vi "RunTest3.vi"(8 "error in (no error)":errorcluster, 11 "Prueba01 in":refnum<class "Prueba01.lvclass">) -> (0 "error out":errorcluster, 2 "resultado":string, 3 "Prueba01 out":refnum<class "Prueba01.lvclass">)   [LabVIEW 2019]
uses:
  Prueba01.lvclass
panel:
  in  "Tab Control":enum32{"externo", "interno"}(tab)
  out "max_tol_ajuste_ext":dbl
  out "Nivel_externo":dbl
  in  "generar":bool
  out "frecuencia":dbl
  out "cumple":bool
  out "no_cumple":bool
  out "frec_ref":dbl
  out "nivel_ref":dbl
  in  "señal_antes_ajuste":dbl
  out "error_ext":dbl
  out "inc_extend":dbl
  in  "seguir":bool
  out "voltaje":dbl
  out "frecuencia 2":dbl
  out "tipo generador":string
  out "max_tol_ajuste_int":dbl
  in  "Nivel_interno":dbl
  out "frecuencia_int":dbl
  out "cumple_int":bool
  out "no_cumple_int":bool
  out "frec_ref_int":dbl
  out "nivel_ref_int":dbl
  in  "señal_antes_ajuste_int":dbl
  out "error_ext_int":dbl
  out "inc_extend_int":dbl
  in  "seguir_int":bool
  out "tipo gen_int":string
  # "Elección Señal de Referencia \nsegún marca y modelo de sonómetro"
  # "Cumple"
  # "No Cumple"
  # "Máxima Tolerancia de Ajuste"
  # "Frecuencia"
  # "Nivel"
  # "Frecuencia Señal de Referencia [Hz]"
  # "Nivel de Señal de Referencia [dB] (a)"
  # "Nivel de señal medida antes de ajuste [dB] (b)"
  # "Error [dB]"
  # "Incertidumbre Expandida ± [dB] (k=2)"
  # "1. Indicación a la frecuencia de comprobación. IEC 61672-3: 2006 Cláusula 9"
  # "Monitoreo"
  # "Frecuencia"
  # "Hz"
  # "Voltaje"
  # "V"
  # "Elección Señal de Referencia \nsegún marca y modelo de sonómetro"
  # "Máxima Tolerancia de ajuste"
  # "Cumple"
  # "No Cumple"
  # "Frecuencia"
  # "Nivel"
  # "Frecuencia Señal de Referencia [Hz]"
  # "Nivel de Señal de Referencia [dB] (a)"
  # "Nivel de señal medida antes de ajuste [dB] (b)"
  # "Error [dB]"
  # "Incertidumbre Expandida ± [dB] (k=2)"
  # "1. Indicación a la frecuencia de comprobación. IEC 61672-3: 2006 Cláusula 9"
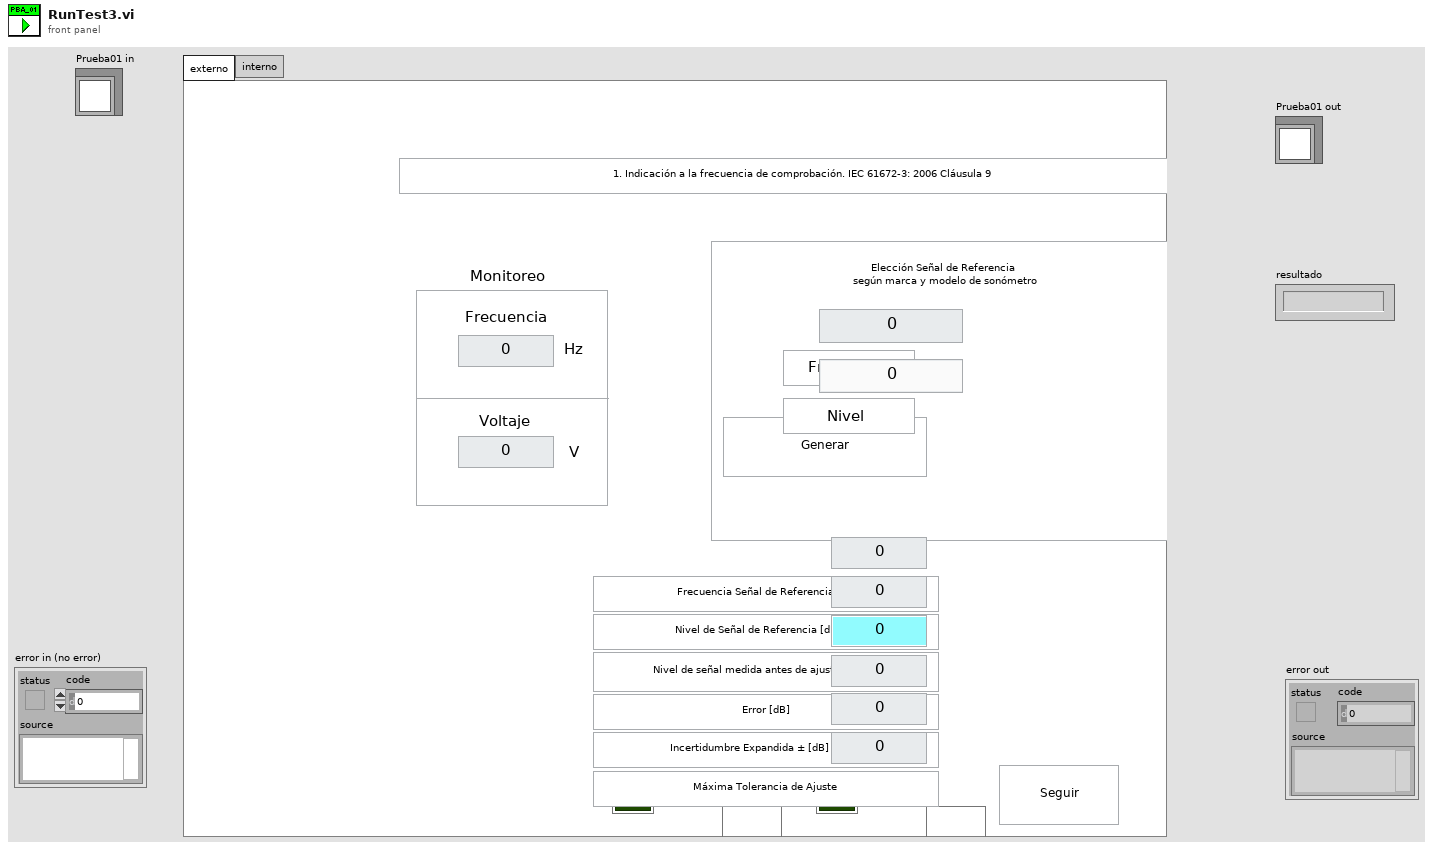
[diagram p1: front panel]
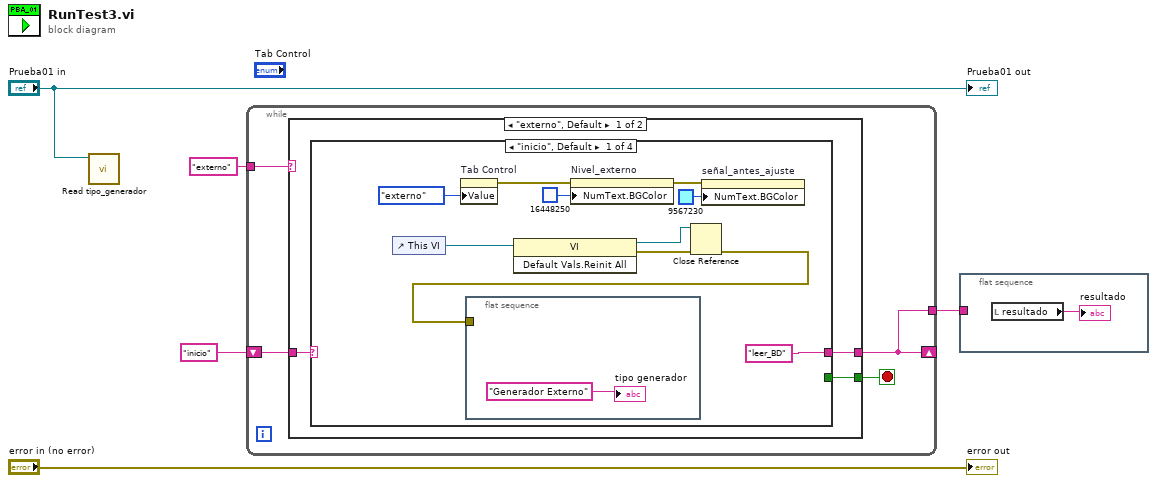
[diagram p0: block diagram]
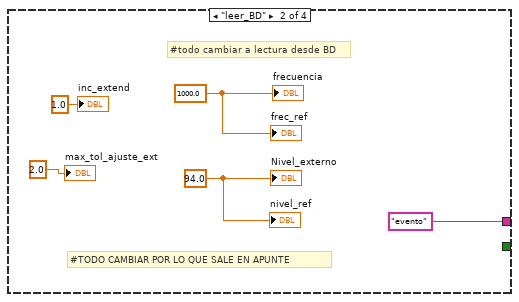
[diagram p2: hidden frame]
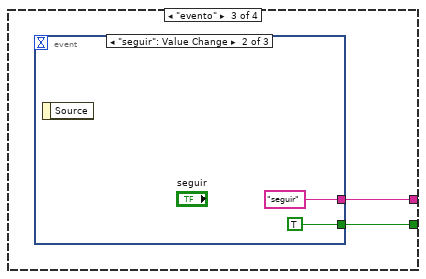
[diagram p3: hidden frame]
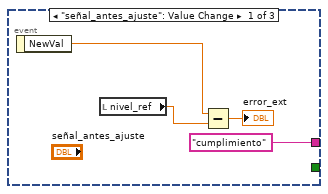
[diagram p4: hidden frame]
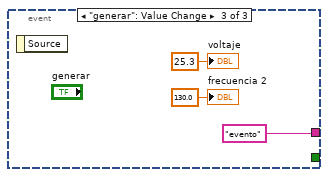
[diagram p5: hidden frame]
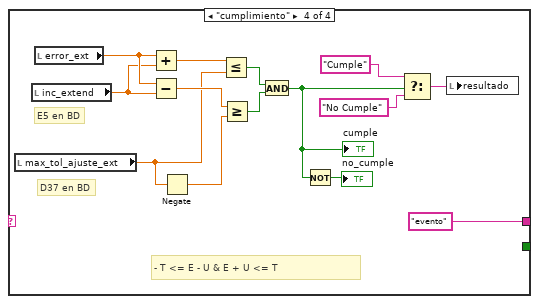
[diagram p6: hidden frame]
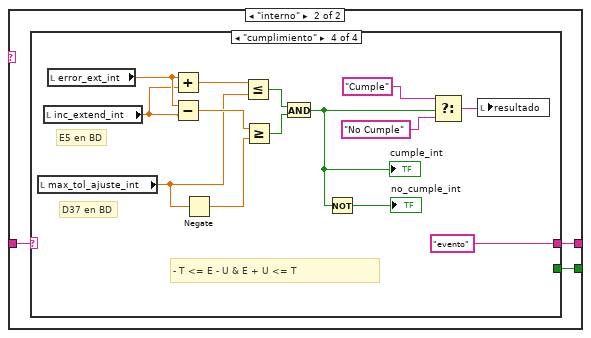
[diagram p7: hidden frame]
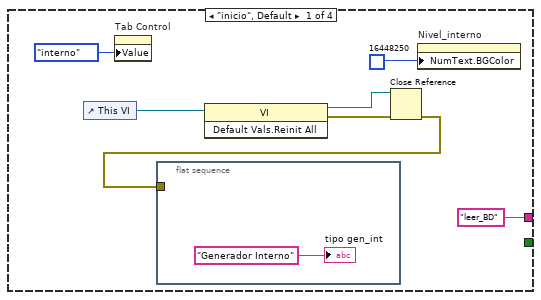
[diagram p8: hidden frame]
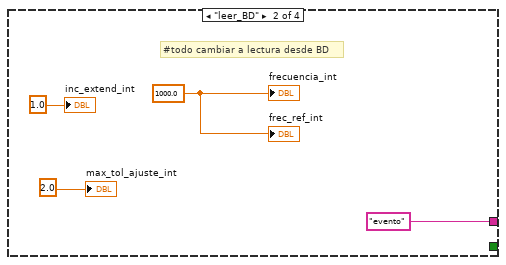
[diagram p9: hidden frame]
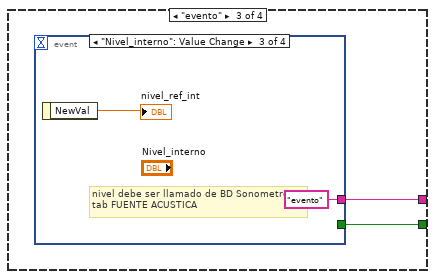
[diagram p10: hidden frame]
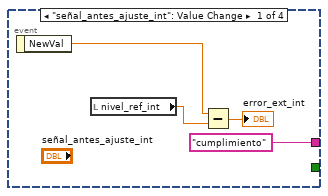
[diagram p11: hidden frame]
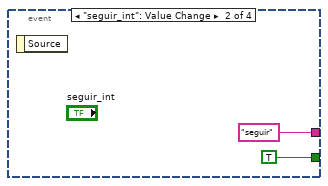
[diagram p12: hidden frame]
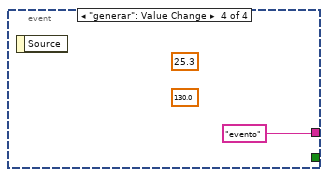
[diagram p13: hidden frame]
diagram:
  n1 = call-dynamic "Read tipo_generador.vi"("Prueba01 in"="Prueba01 in") -> ()  [unwired: 8 in, 3 out]
  n2 = while {
    shift-right: [w6] -> _
    shift-left: "inicio" -> [w9]
    tunnel: "externo" ("tipo_generador") -> [w7]
    tunnel: [w6] -> w2
    stop <- w8 stop-if-true
    n3 = case shown="\"externo\", Default" w7 {
      tunnel: w9 -> [w12 w56]
      tunnel: [w11 w55] -> w8
      tunnel: [w10 w54] -> w6
      frame "externo", Default {
        n4 = case shown="\"inicio\", Default" w12 {
          tunnel: ["leer_BD" "evento" w30 "evento"] -> w10
          tunnel: [_ _ w29 _] -> w11
          frame "inicio", Default {
            n5 = control-ref of="This VI"() -> (w20:refnum<vi>)
            n6 = property on="Tab Control" class="TabCtl (strict)"("Value"=enum32{"externo", "interno"}."externo" ("Tab Control")) -> (error out=w15:errorcluster)  [unwired: 2 in, 1 out]
            n7 = flat-sequence {
              tunnel: w18 -> [_]
              frame #0 {
                "tipo generador" <- "Generador Externo" ("Generador")
              }
            }
            n8 = invoke class="VI" method="Default Vals.Reinit All"(reference=w20) -> (reference out=w21:refnum<vi>, error out=w22:errorcluster)  [unwired: 2 in, 1 out]
            n9 = property on="Nivel_externo" class="DigNum (strict)"(error in=w15, "NumText.BGColor"=u32 16448250) -> (error out=w14:errorcluster)  [unwired: 1 in, 1 out]
            n10 = Close Reference(reference=w21, error in (no error)=w22) -> (error out=w18:errorcluster)
            n11 = property on="señal_antes_ajuste" class="DigNum (strict)"(error in=w14, "NumText.BGColor"=u32 9567230) -> ()  [unwired: 1 in, 2 out]
          }
          frame "leer_BD" {
            w26 = 94.0 ("Nivel_externo")
            w27 = 1000.0 ("frecuencia")
            # "#TODO CAMBIAR POR LO QUE SALE EN APUNTE"
            # "#todo cambiar a lectura desde BD"
            "frecuencia" <- w27
            "frec_ref" <- w27
            "Nivel_externo" <- w26
            "nivel_ref" <- w26
            "inc_extend" <- 1.0 ("incertidumbre")
            "max_tol_ajuste_ext" <- 2.0 ("Tolerancia")
          }
          frame "evento" {
            n12 = event shown="[1] \"seguir\": Value Change" {
              selector: _ -> [_ _ _]
              dyn-events: _ -> [_ _ _]
              timeout: _ -> [_ _ _]
              tunnel: ["cumplimiento" "seguir" "evento"] -> w30
              tunnel: [_ TRUE _] -> w29
              event "señal_antes_ajuste": Value Change {
                n13 = event-data() -> ("NewVal"=w32:dbl)  [unwired: 1 in]
                n14 = local read "nivel_ref"() -> (w31:dbl)
                n15 = Subtract(x=w32, y=w31) -> (x-y=→"error_ext":dbl)
              }
              event "seguir": Value Change {
                n16 = event-data() -> ()  [unwired: 1 in, 1 out]
              }
              event "generar": Value Change {
                n17 = event-data() -> ()  [unwired: 1 in, 1 out]
                "frecuencia 2" <- 130.0 ("frecuencia")
                "voltaje" <- 25.3 ("voltaje")
              }
            }
          }
          frame "cumplimiento" {
            # "D37 en BD"
            # "- T <= E - U & E + U <= T"
            # "E5 en BD"
            n18 = local read "max_tol_ajuste_ext"() -> (w40:dbl)
            n19 = local read "inc_extend"() -> (w43:dbl)
            n20 = local read "error_ext"() -> (w49:dbl)
            n21 = Add(x=w49, y=w43) -> (x+y=w48:dbl)
            n22 = Subtract(x=w49, y=w43) -> (x-y=w45:dbl)
            n23 = Negate(x=w40) -> (-x=w42:dbl)
            n24 = Less Or Equal?(x=w48, y=w40) -> (x <= y?=w47:bool)
            n25 = Greater Or Equal?(x=w45, y=w42) -> (x >= y?=w46:bool)
            n26 = And(x=w47, y=w46) -> (x .and. y?=w44:bool)
            "cumple" <- w44
            n27 = Not(x=w44) -> (.not. x?=→"no_cumple":bool)
            n28 = Select(t="Cumple", s=w44, f="No Cumple") -> (s? t:f=w41:string)
            n29 = local write "resultado"(w41) -> ()
          }
        }
      }
      frame "interno" {
        n30 = case shown="\"cumplimiento\"" w56 {
          tunnel: ["leer_BD" "evento" w70 "evento"] -> w54
          tunnel: [_ _ w69 _] -> w55
          frame "inicio", Default {
            n31 = control-ref of="This VI"() -> (w61:refnum<vi>)
            n32 = property on="Tab Control" class="TabCtl (strict)"("Value"=enum32{"externo", "interno"}."interno" ("Tab Control")) -> ()  [unwired: 2 in, 2 out]
            n33 = flat-sequence {
              tunnel: w59 -> [_]
              frame #0 {
                "tipo gen_int" <- "Generador Interno" ("Generador")
              }
            }
            n34 = invoke class="VI" method="Default Vals.Reinit All"(reference=w61) -> (reference out=w62:refnum<vi>, error out=w63:errorcluster)  [unwired: 2 in, 1 out]
            n35 = Close Reference(reference=w62, error in (no error)=w63) -> (error out=w59:errorcluster)
            n36 = property on="Nivel_interno" class="DigNum (strict)"("NumText.BGColor"=u32 16448250) -> ()  [unwired: 2 in, 2 out]
          }
          frame "leer_BD" {
            w67 = 1000.0 ("frecuencia")
            # "#todo cambiar a lectura desde BD"
            "frecuencia_int" <- w67
            "frec_ref_int" <- w67
            "inc_extend_int" <- 1.0 ("incertidumbre")
            "max_tol_ajuste_int" <- 2.0 ("Tolerancia")
          }
          frame "evento" {
            n37 = event shown="[2] \"Nivel_interno\": Value Change" {
              selector: _ -> [_ _ _ _]
              dyn-events: _ -> [_ _ _ _]
              timeout: _ -> [_ _ _ _]
              tunnel: ["cumplimiento" "seguir" "evento" "evento"] -> w70
              tunnel: [_ TRUE _ _] -> w69
              event "señal_antes_ajuste_int": Value Change {
                n38 = event-data() -> ("NewVal"=w73:dbl)  [unwired: 1 in]
                n39 = local read "nivel_ref_int"() -> (w72:dbl)
                n40 = Subtract(x=w73, y=w72) -> (x-y=→"error_ext_int":dbl)
              }
              event "seguir_int": Value Change {
                n41 = event-data() -> ()  [unwired: 1 in, 1 out]
              }
              event "Nivel_interno": Value Change {
                # "nivel debe ser llamado de BD Sonometro\ntab FUENTE ACUSTICA"
                n42 = event-data() -> ("NewVal"=→"nivel_ref_int":dbl)  [unwired: 1 in]
              }
              event "generar": Value Change {
                (unwired) 130.0 ("frecuencia")
                (unwired) 25.3 ("voltaje")
                n43 = event-data() -> ()  [unwired: 1 in, 1 out]
              }
            }
          }
          frame "cumplimiento" {
            # "D37 en BD"
            # "- T <= E - U & E + U <= T"
            # "E5 en BD"
            n44 = local read "max_tol_ajuste_int"() -> (w80:dbl)
            n45 = local read "inc_extend_int"() -> (w83:dbl)
            n46 = local read "error_ext_int"() -> (w84:dbl)
            n47 = Add(x=w84, y=w83) -> (x+y=w90:dbl)
            n48 = Subtract(x=w84, y=w83) -> (x-y=w87:dbl)
            n49 = Negate(x=w80) -> (-x=w86:dbl)
            n50 = Less Or Equal?(x=w90, y=w80) -> (x <= y?=w89:bool)
            n51 = Greater Or Equal?(x=w87, y=w86) -> (x >= y?=w88:bool)
            n52 = And(x=w89, y=w88) -> (x .and. y?=w82:bool)
            "cumple_int" <- w82
            n53 = Not(x=w82) -> (.not. x?=→"no_cumple_int":bool)
            n54 = Select(t="Cumple", s=w82, f="No Cumple") -> (s? t:f=w85:string)
            n55 = local write "resultado"(w85) -> ()
          }
        }
      }
    }
  }
  n56 = flat-sequence {
    tunnel: w2 -> [_]
    frame #0 {
      n57 = local read "resultado"() -> (→"resultado":string)
    }
  }
  "error out" <- "error in (no error)"
  "Prueba01 out" <- "Prueba01 in"
